vi "Update UI.vi"(8 "error in (no error)":errorcluster, 10 "DataExchange":T1, 11 "Microscope Controller in":refnum<class "MicroscopeController.lvclass">) -> (0 "error out":errorcluster, 3 "Microscope Controller out":refnum<class "MicroscopeController.lvclass">)   [LabVIEW 2020, in "MicroscopeController.lvlib" / "MicroscopeController.lvclass"]
uses:
  MicroscopeController.lvclass
  Model/Hardware Abstraction Layer/Component/Device/Device/DataExchange.ctl
  MicroscopeController.lvclass/MicroscopeController.ctl
  Interface/DataListener/DataListener.lvclass
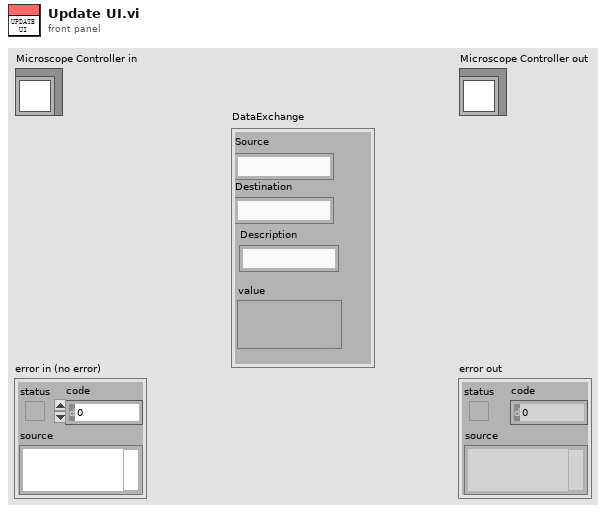
[diagram p1: front panel]
types:
  T1 = typedef "DataListener.lvclass/DataExchange.ctl" = cluster{"Source":string, "Destination":string, "Description":string, "value":variant}
  T2 = enum32{"Invalid", "Standard", "Closed", "Hidden", "Minimized", "Maximized"}
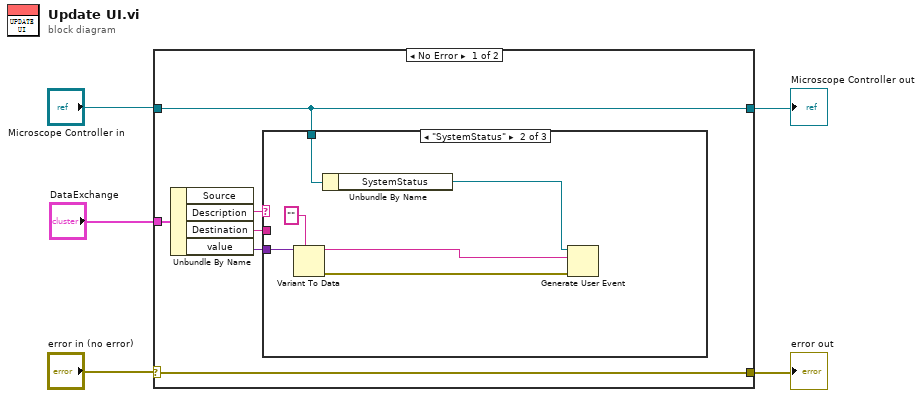
[diagram p0: block diagram]
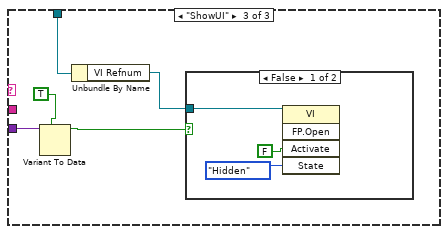
[diagram p3: hidden frame]
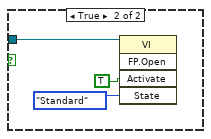
[diagram p4: hidden frame]
diagram:
  n1 = case shown="No Error" "error in (no error)" {
    selector: "error in (no error)" -> [w11 w30]
    tunnel: [w11 w30] -> w2
    tunnel: [w6 w29] -> w4
    tunnel: "Microscope Controller in" -> [w6 w29]
    tunnel: "DataExchange" -> [w10 _]
    frame No Error {
      n2 = Unbundle By Name(w10) -> ("Description"=w7:string, "Destination"=w8:string, "value"=w9:variant)  [unwired: 1 out]
      n3 = case shown="\"SystemStatus\"" w7 {
        tunnel: w9 -> [_ w17 w22]
        tunnel: w8 -> [_ _ _]
        tunnel: w6 -> [_ w16 w21]
        frame Default {
        }
        frame "SystemStatus" {
          n4 = Variant To Data(type="" ("event data"), Variant=w17) -> (data=w12:string, error out=w14:errorcluster)  [unwired: 1 in]
          n5 = Unbundle By Name(w16) -> ("SystemStatus"=w15:refnum<user-event>)
          n6 = Generate User Event(user event=w15, event data cluster=w12, error in=w14) -> ()  [unwired: 1 in, 2 out]
        }
        frame "ShowUI" {
          n7 = Variant To Data(type=TRUE, Variant=w22) -> (data=w19:bool)  [unwired: 1 in, 1 out]
          n8 = Unbundle By Name(w21) -> ("VI Refnum"=w18:refnum<vi>)
          n9 = case shown="False" w19 {
            tunnel: w18 -> [w25 w28]
            frame False {
              n10 = invoke class="VI" method="FP.Open"(reference=w25, "Activate"=FALSE ("Activate?"), "State"=T2."Hidden") -> ()  [unwired: 2 in, 5 out]
            }
            frame True {
              n11 = invoke class="VI" method="FP.Open"(reference=w28, "Activate"=TRUE ("Activate?"), "State"=T2."Standard") -> ()  [unwired: 2 in, 5 out]
            }
          }
        }
      }
    }
    frame Error {
    }
  }
  "error out" <- w2
  "Microscope Controller out" <- w4
